vi "ReadPowerState.vi"(8 "error in (no error)":errorcluster, 11 "Stereo in":refnum<class "Stereo.lvclass">) -> (0 "error out":errorcluster, 2 "PowerState":bool, 3 "Stereo out":refnum<class "Stereo.lvclass">)   [LabVIEW 2013, in "Stereo.lvclass"]
uses:
  Stereo.lvclass
  Stereo.lvclass/Stereo.ctl
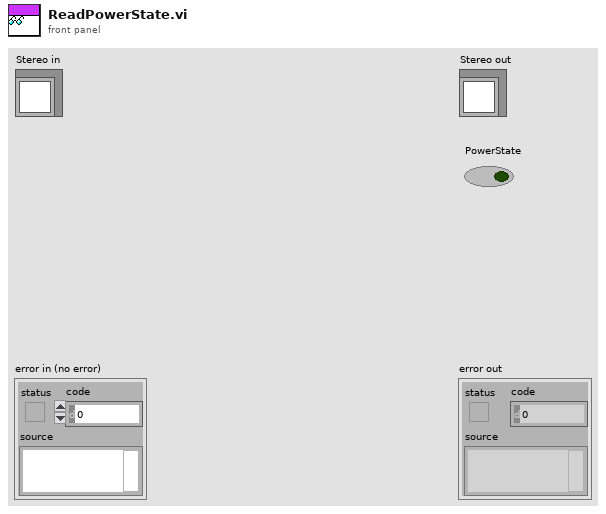
[diagram p1: front panel]
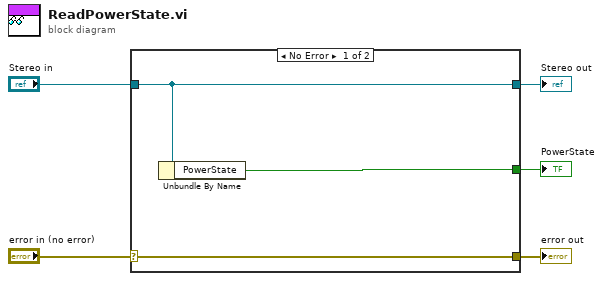
[diagram p0: block diagram]
diagram:
  n1 = case shown="No Error" "error in (no error)" {
    selector: "error in (no error)" -> [w8 w9]
    tunnel: [w8 w9] -> w4
    tunnel: [w7 w10] -> w2
    tunnel: "Stereo in" -> [w7 w10]
    tunnel: [w6 _] -> w1
    frame No Error {
      n2 = Unbundle By Name(w7) -> ("PowerState"=w6:bool)
    }
    frame Error {
    }
  }
  "error out" <- w4
  "Stereo out" <- w2
  "PowerState" <- w1
